vi "Write Byte.vi"(7 "Mode (0)":u8, 8 "error in (no error)":errorcluster, 9 "Value":u8 format="%.0b", 10 "VISA resource name in":refnum<visa-resource-name>, 11 "LCD-I2C in":refnum<class "LCD-I2C.lvclass">) -> (0 "error out":errorcluster, 2 "VISA resource name":refnum<visa-resource-name>, 3 "LCD-I2C out":refnum<class "LCD-I2C.lvclass">)   [LabVIEW 2020, in "CTI-Visa-DeviceLib.lvlib" / "LCD-I2C.lvclass"]
uses:
  LCD-I2C.lvclass
  LCD-I2C.lvclass/LCD-I2C.ctl
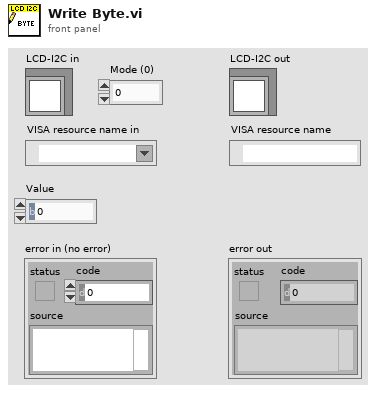
[diagram p1: front panel]
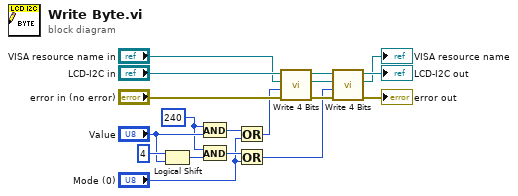
[diagram p0: block diagram]
diagram:
  w14 = u8 240 ("y")
  n1 = Logical Shift(y=i16 4, x="Value") -> (x << y=w15:u8)
  n2 = And(x=w14, y="Value") -> (x .and. y?=w13:u8)
  n3 = And(x=w14, y=w15) -> (x .and. y?=w12:u8)
  n4 = Or(x=w13, y="Mode (0)") -> (x .or. y?=w5:u8)
  n5 = Or(x=w12, y="Mode (0)") -> (x .or. y?=w4:u8)
  n6 = call "Write 4 Bits.vi"("error in (no error)"="error in (no error)", "Value"=w5, "VISA resource name in"="VISA resource name in", "LCD-I2C in"="LCD-I2C in") -> ("error out"=w10:errorcluster, "VISA resource name"=w3:refnum<visa-resource-name>, "LCD-I2C out"=w7:refnum<class "LCD-I2C.lvclass">)  [unwired: 5 in]
  n7 = call "Write 4 Bits.vi"("error in (no error)"=w10, "Value"=w4, "VISA resource name in"=w3, "LCD-I2C in"=w7) -> ("error out"=→"error out":errorcluster, "VISA resource name"=→"VISA resource name":refnum<visa-resource-name>, "LCD-I2C out"=→"LCD-I2C out":refnum<class "LCD-I2C.lvclass">)  [unwired: 5 in]
